vi "Get All Panels.vi"(8 "error in (no error)":errorcluster, 11 "PanelArray in":refnum<class "ArrayManager.lvclass">) -> (0 "error out":errorcluster, 2 "Panels":refnum<class "ArrayPanel.lvclass">[](array[class]), 3 "PanelArray out":refnum<class "ArrayManager.lvclass">)   [LabVIEW 2020, in "OOPanel.lvlib" / "ArrayManager.lvclass"]
uses:
  ArrayManager.lvclass
  ArrayPanel/ArrayPanel.lvclass
  ArrayManager.lvclass/ArrayManager.ctl
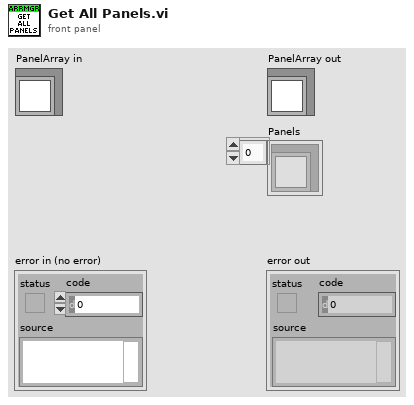
[diagram p1: front panel]
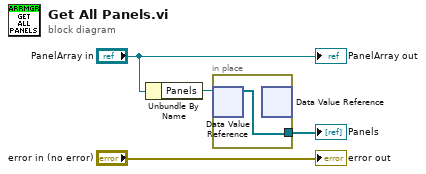
[diagram p0: block diagram]
diagram:
  n1 = Unbundle By Name("PanelArray in") -> ("Panels"=w3:refnum<data-value>)
  n2 = in-place {
    in-place-border: [w5] -> w1
    n3 = in-place-dvr #1(w3) -> (w5:refnum<class "ArrayPanel.lvclass">[])  [unwired: 1 out]
    n4 = in-place-dvr #1() -> ()  [unwired: 1 in, 2 out]
  }
  "Panels" <- w1
  "error out" <- "error in (no error)"
  "PanelArray out" <- "PanelArray in"
